vi "Updated Shot.vi"(11 "One Button\nShot":bool) -> ()   [LabVIEW 2019, in "8085 VI Library.lvlib"]
uses:
  8085 VI Library.lvlib
  <vilib>/Rock Robotics/WPI/ThirdParty/Phoenix-LabVIEW/Motor Controller/Controls/CTRE_Phoenix_MotorControl_ControlMode.ctl
panel:
  in  "Output":T1 items=["PercentOutput"=0, "Position"=1, "Velocity"=2, "Current"=3, "Follower"=5, "MotionProfile"=6, "MotionMagic"=7, "MotionProfileArc"=10, "Disabled"=15]
  in  "Output 5":T1 items=["PercentOutput"=0, "Position"=1, "Velocity"=2, "Current"=3, "Follower"=5, "MotionProfile"=6, "MotionMagic"=7, "MotionProfileArc"=10, "Disabled"=15]
  in  "Intake 4":T1 items=["PercentOutput"=0, "Position"=1, "Velocity"=2, "Current"=3, "Follower"=5, "MotionProfile"=6, "MotionMagic"=7, "MotionProfileArc"=10, "Disabled"=15]
  in  "Control Mode 7":T1 items=["PercentOutput"=0, "Position"=1, "Velocity"=2, "Current"=3, "Follower"=5, "MotionProfile"=6, "MotionMagic"=7, "MotionProfileArc"=10, "Disabled"=15]
  out "Trigger \nSqueeze On":bool
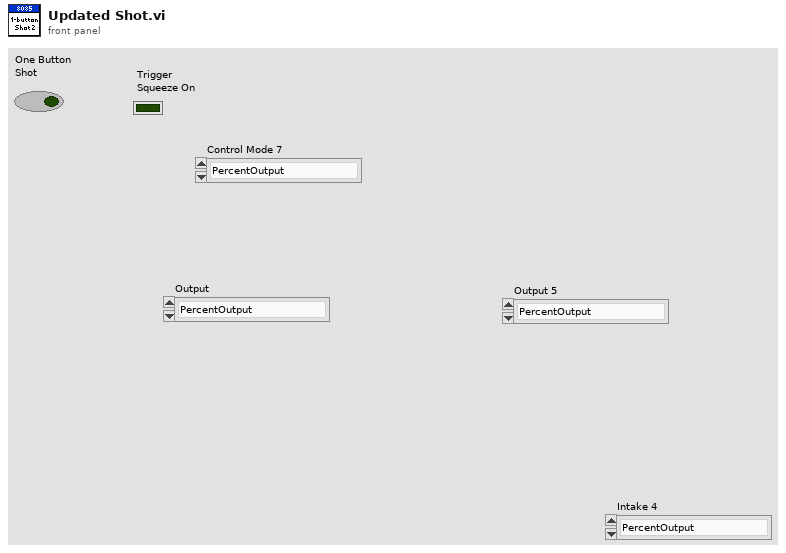
[diagram p1: front panel]
types:
  T1 = typedef "CTRE_Phoenix_MotorControl_ControlMode.ctl" = u16
  T2 = typedef "WPI_MotorControlDeviceRef.ctl" = cluster{"DeviceStatus":errorcluster, "Type":T3, "PWM":cluster{"PWM Channel":T4, "DeadBand":T5}, "CAN":cluster{"Device Number":u8, "SetOutput VI Ref":variant, "GetOutput VI Ref":variant, "Enable VI Ref":variant, "Disable VI Ref":variant, "Data":variant}, "Invert":bool, "DIO PWM":cluster{"PWM \"Enable\" Channel":T4, "DIOChannel":T6, "PWM Rate":dbl}}
  T3 = typedef "WPI_MotorControlType.ctl" = enum16{"PWM", "CAN", "DIO PWM"}
  T4 = typedef "FPGA_DIOPWMChannel.ctl" = enum8{"PWM 0", "PWM 1", "PWM 2", "PWM 3", "PWM 4", "PWM 5", "PWM 6", "PWM 7", "PWM 8", "PWM 9", "PWM MXP 0", "PWM MXP 1", "PWM MXP 2", "PWM MXP 3", "PWM MXP 4", "PWM MXP 5", "PWM MXP 6", "PWM MXP 7", "PWM MXP 8", "PWM MXP 9", "Invalid"}
  T5 = typedef "WPI_PWMDeadband.ctl" = cluster{"Name":string, "maxPositivePwm":i32, "minPositivePwm":i32, "centerPwm":i32, "maxNegativePwm":i32, "minNegativePwm":i32, "angularRange":u16}
  T6 = typedef "FPGA_DIOChannel.ctl" = enum8{"DIO 0", "DIO 1", "DIO 2", "DIO 3", "DIO 4", "DIO 5", "DIO 6", "DIO 7", "DIO 8", "DIO 9", "DIO MXP 0", "DIO MXP 1", "DIO MXP 2", "DIO MXP 3", "DIO MXP 4", "DIO MXP 5", "DIO MXP 6", "DIO MXP 7", "DIO MXP 8", "DIO MXP 9", "DIO MXP 10", "DIO MXP 11", "DIO MXP 12", "DIO MXP 13", "DIO MXP 14", "DIO MXP 15", "SPI Port CS1", "SPI Port CS2", "SPI Port CS3", "SPI Port MISO", "SPI Port MOSI", "Invalid"}
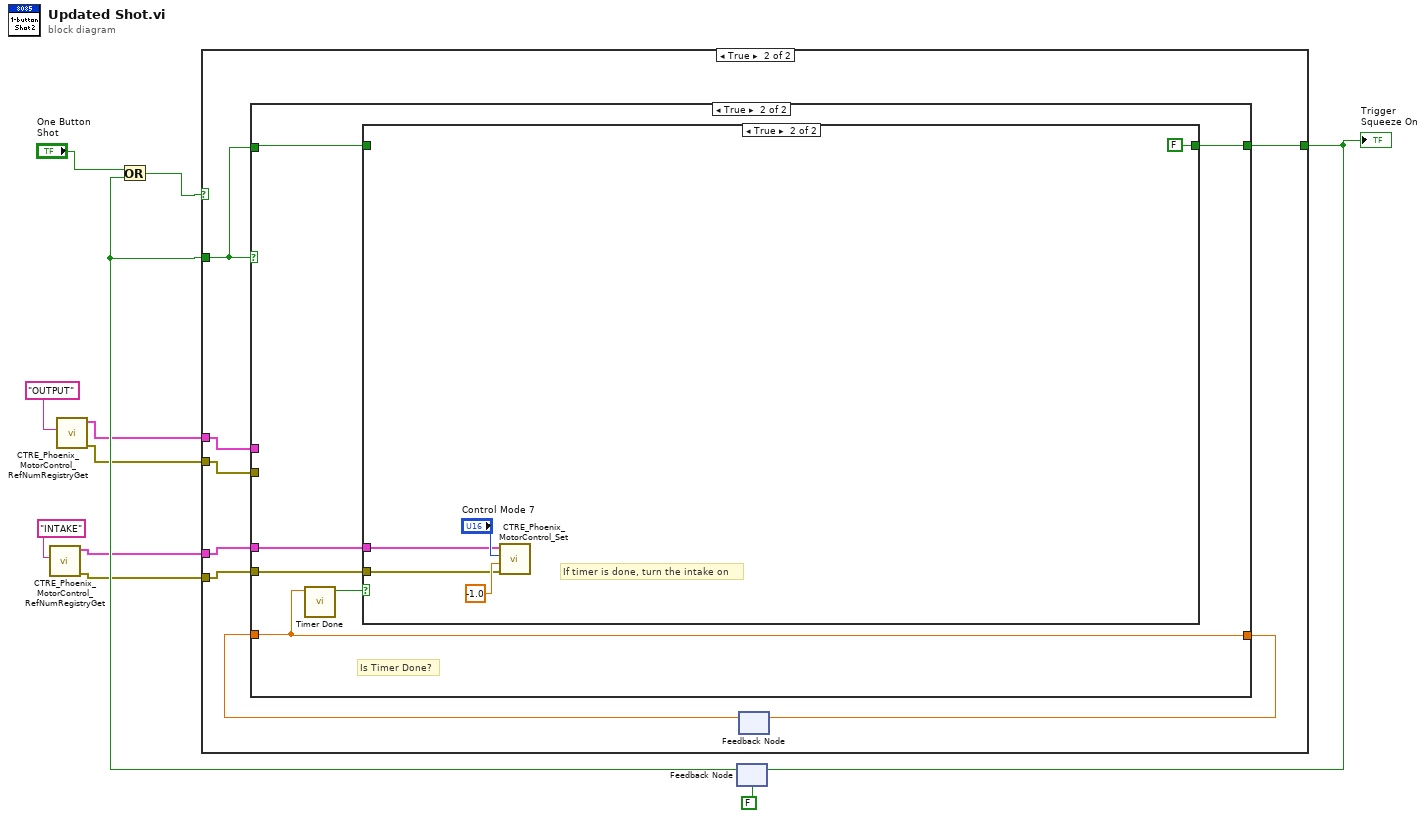
[diagram p0: block diagram]
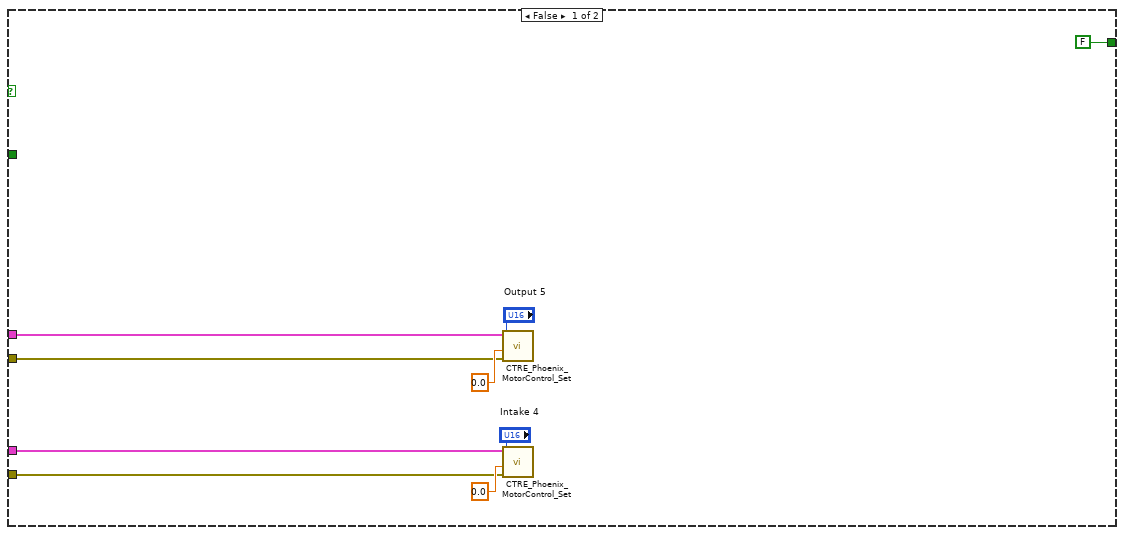
[diagram p2: hidden frame]
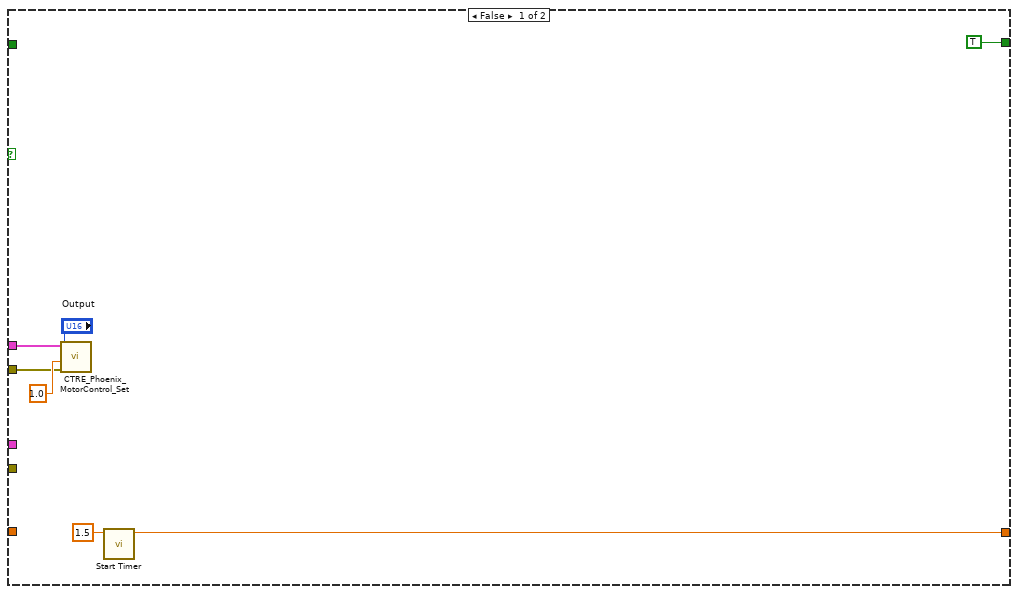
[diagram p3: hidden frame]
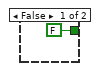
[diagram p4: hidden frame]
diagram:
  n1 = call <vilib>:"CTRE_Phoenix_MotorControl_RefNumRegistryGet.vi"("refnum name"="INTAKE") -> ("error out"=w1:errorcluster, "PhoenixMotorControlDevRef"=w2:T2)  [unwired: 9 in]
  n2 = call <vilib>:"CTRE_Phoenix_MotorControl_RefNumRegistryGet.vi"("refnum name"="OUTPUT") -> ("error out"=w3:errorcluster, "PhoenixMotorControlDevRef"=w4:T2)  [unwired: 9 in]
  n3 = feedback #1(FALSE) -> (w9:bool)
  n4 = Or(x="One Button\nShot", y=w9) -> (x .or. y?=w10:bool)
  n5 = case shown="True" w10 {
    tunnel: w9 -> [_ w25]
    tunnel: [FALSE w26] -> w8
    tunnel: w4 -> [w15 w24]
    tunnel: w3 -> [w14 w23]
    tunnel: w2 -> [w13 w22]
    tunnel: w1 -> [w12 w21]
    frame False {
      n6 = call <vilib>:"CTRE_Phoenix_MotorControl_Set.vi"("error in (no error)"=w14, "Output"=0.0, "Control Mode"="Output 5", "PhoenixMotorControlDevRef"=w15) -> ()  [unwired: 6 in, 2 out]
      n7 = call <vilib>:"CTRE_Phoenix_MotorControl_Set.vi"("error in (no error)"=w12, "Output"=0.0, "Control Mode"="Intake 4", "PhoenixMotorControlDevRef"=w13) -> ()  [unwired: 6 in, 2 out]
    }
    frame True {
      n8 = feedback #2() -> (w27:dbl)  [unwired: 1 in]
      n9 = case shown="True" w25 {
        tunnel: [w34 w38] -> w28
        tunnel: w27 -> [_ w38]
        tunnel: [TRUE w41] -> w26
        tunnel: w25 -> [_ w40]
        tunnel: w24 -> [w30 _]
        tunnel: w23 -> [w29 _]
        tunnel: w22 -> [_ w37]
        tunnel: w21 -> [_ w36]
        frame False {
          n10 = call <vilib>:"CTRE_Phoenix_MotorControl_Set.vi"("error in (no error)"=w29, "Output"=1.0, "Control Mode"="Output", "PhoenixMotorControlDevRef"=w30) -> ()  [unwired: 6 in, 2 out]
          n11 = call "Start Timer.vi"("Wait\nTime"=1.5 ("Wait\nTime")) -> ("Elapsed Time"=w34:dbl)  [unwired: 10 in]
        }
        frame True {
          # "Is Timer Done?"
          n12 = call "Timer Done.vi"("Wait\nTime"=w38) -> ("Timer \nDone?"=w39:bool)  [unwired: 10 in]
          n13 = case shown="True" w39 {
            tunnel: [FALSE FALSE] -> w41
            tunnel: w40 -> [_ _]
            tunnel: w37 -> [_ w45]
            tunnel: w36 -> [_ w44]
            frame False {
            }
            frame True {
              # "If timer is done, turn the intake on"
              n14 = call <vilib>:"CTRE_Phoenix_MotorControl_Set.vi"("error in (no error)"=w44, "Output"=-1.0, "Control Mode"="Control Mode 7", "PhoenixMotorControlDevRef"=w45) -> ()  [unwired: 6 in, 2 out]
            }
          }
        }
      }
      n15 = feedback-in #2(w28) -> ()
    }
  }
  "Trigger \nSqueeze On" <- w8
  n16 = feedback-in #1(w8) -> ()
